vi "写入当前抽取数据数组.vi"(8 "error in (no error)":errorcluster caption="错误输入（无错误）", 11 "抽取参数输入":refnum<class "抽取参数.lvclass">) -> (0 "error out":errorcluster caption="错误输出", 3 "抽取参数输出":refnum<class "抽取参数.lvclass">)   [LabVIEW 2020, in "抽取参数.lvclass"]
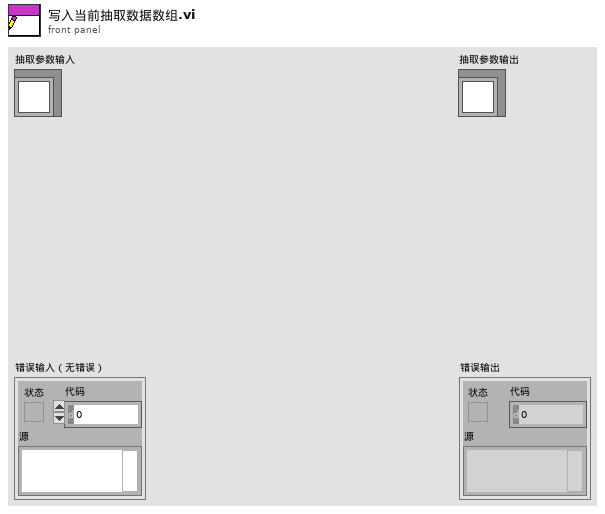
[diagram p1: front panel]
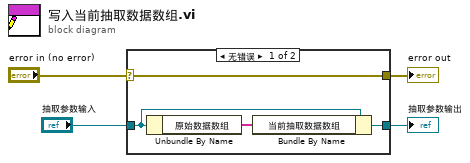
[diagram p0: block diagram]
diagram:
  n1 = case shown="无错误" "error in (no error)" {
    selector: "error in (no error)" -> [w8 w9]
    tunnel: [w8 w9] -> w3
    tunnel: [w7 w10] -> w1
    tunnel: "抽取参数输入" -> [w6 w10]
    frame No Error {
      n2 = Unbundle By Name(w6) -> ("原始数据数组"=w5:string[])
      n3 = Bundle By Name(cluster=w6, "当前抽取数据数组"=w5) -> (w7:refnum<class "抽取参数.lvclass">)
    }
    frame Error {
    }
  }
  "error out" <- w3
  "抽取参数输出" <- w1
